vi "Normalize String Length.vi"(9 "Fill with":string, 10 "Length":i32=25, 11 "String in":string) -> (3 "Normalized String":string)   [LabVIEW 2025]
doc: "This VI normalizes the length of an array to the specified length by adding the character specified in the \"Fill with\" input (Default: space)."
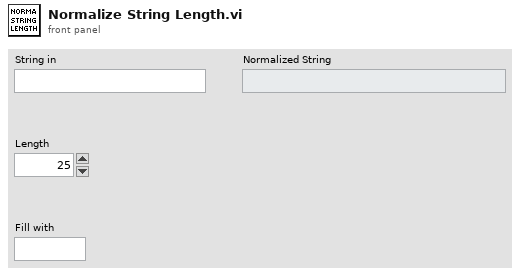
[diagram p1: front panel]
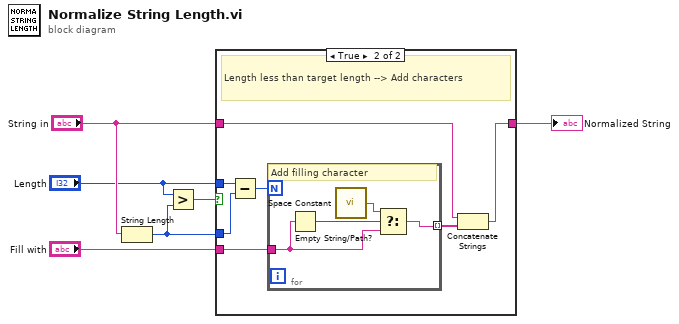
[diagram p0: block diagram]
diagram:
  n1 = String Length(string="String in") -> (length=w1:i32)
  n2 = Greater?(x="Length", y=w1) -> (0:w6:bool)
  n3 = case shown="True" w6 {
    tunnel: "String in" -> [w7 w11]
    tunnel: "Length" -> [_ w14]
    tunnel: w1 -> [_ w13]
    tunnel: [w7 w9] -> w4
    tunnel: "Fill with" -> [_ w8]
    frame False {
      # "String is equal or longer than specified length"
    }
    frame True {
      # "Length less than target length --> Add characters"
      n4 = Subtract(x=w14, y=w13) -> (x-y=w12:i32)
      n5 = for {
        N: w12 -> [_]
        tunnel: [w15] -> w10 mode=indexing
        tunnel: w8 -> [w16]
        # "Add filling character"
        n6 = Empty String/Path?(string/path=w16) -> (empty?=w18:bool)
        n7 = call <vilib>:"Space Constant.vi"() -> ("String"=w17:string)
        n8 = Select(t=w17, s=w18, f=w16) -> (s? t:f=w15:string)
      }
      n9 = Concatenate Strings(w11, w10) -> (w9:string)
    }
  }
  "Normalized String" <- w4
